vi "NI VeriStand - Run Project.vi"(8 "error in (no error)":errorcluster, 10 "Show Progress (F)":bool, 11 "Project Ref in":T1) -> (0 "error out":errorcluster, 3 "Project Ref out":T1)   [LabVIEW 2020, in "NI_VS Project ExecutionAPI.lvlib"]
doc: "Runs an NI VeriStand project."
uses:
  <vilib>/NI VeriStand/Execution/Project/NI_VS Project ExecutionAPI.lvlib
  <vilib>/NI VeriStand/Execution/Project/Project Ref.ctl
  NationalInstruments.VeriStand.ClientAPI
  NationalInstruments.VeriStand
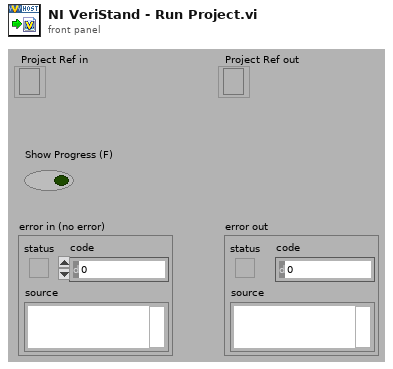
[diagram p1: front panel]
types:
  T1 = typedef "NI_VS Project ExecutionAPI.lvlib/Project Ref.ctl" = refnum<k24>
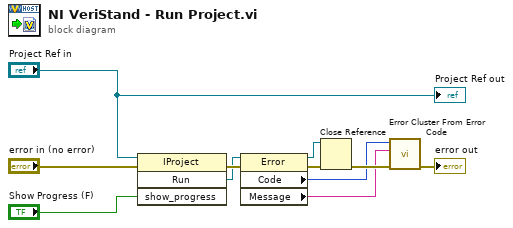
[diagram p0: block diagram]
diagram:
  n1 = invoke class="IProject" method="Run"(reference="Project Ref in", error in="error in (no error)", "show_progress"="Show Progress (F)") -> (error out=w9:errorcluster, "Run"=w4:refnum<k24>)  [unwired: 1 in, 2 out]
  n2 = property class="Error"(reference=w4, error in=w9) -> (reference out=w7:refnum<k24>, error out=w8:errorcluster, "Code"=w3:u32, "Message"=w2:string)
  n3 = Close Reference(reference=w7, error in (no error)=w8) -> (error out=w6:errorcluster)
  n4 = call <vilib>:"Error Cluster From Error Code.vi"("error in (no error)"=w6, "error message (\"\")"=w2, "error code (0)"=w3) -> ("error out"=→"error out":errorcluster)  [unwired: 6 in]
  "Project Ref out" <- "Project Ref in"
